vi "Read DAQ Parameters.vi"(8 "error in (no error)":errorcluster, 11 "DAQ Class in":refnum<class "DAQ Class.lvclass">) -> (0 "error out":errorcluster, 2 "DAQ Parameters":T1, 3 "DAQ Class out":refnum<class "DAQ Class.lvclass">)   [LabVIEW 2014, in "DAQ Class.lvclass"]
uses:
  DAQ Class.lvclass
  DAQ Parameters.ctl
  Trigger Source.ctl
  Trigger Slope.ctl
  Type Defs/OCT DAQ Channel Data Type.ctl
  Clock Control.ctl
  DAQ Class.lvclass/DAQ Class.ctl
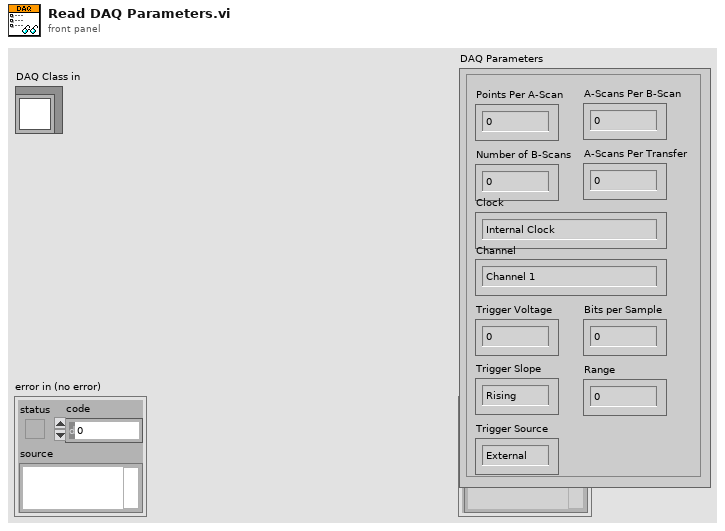
[diagram p1: front panel]
types:
  T1 = typedef "DAQ Class.lvclass/DAQ Parameters.ctl" = cluster{"Points Per A-Scan":u32, "A-Scans Per B-Scan":u32, "Number of B-Scans":u32, "A-Scans Per Transfer":u32, "Trigger Voltage":sgl, "Trigger Source":T2, "Trigger Slope":T3, "Channel":T4, "Clock":T5, "Bits per Sample":dbl, "Range":dbl}
  T2 = typedef "DAQ Class.lvclass/Trigger Source.ctl" = enum16{"External", "Channel A", "Channel B"}
  T3 = typedef "DAQ Class.lvclass/Trigger Slope.ctl" = enum16{"Rising", "Falling"}
  T4 = typedef "OCT DAQ Channel Data Type.ctl" = enum16{"Channel 1", "Channel 2", "Channel 1 and 2"}
  T5 = typedef "DAQ Class.lvclass/Clock Control.ctl" = enum16{"Internal Clock", "External Clock"}
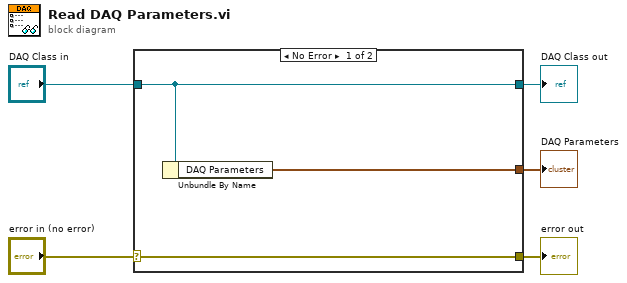
[diagram p0: block diagram]
diagram:
  n1 = case shown="No Error" "error in (no error)" {
    selector: "error in (no error)" -> [w8 w9]
    tunnel: [w8 w9] -> w4
    tunnel: [w7 w10] -> w2
    tunnel: "DAQ Class in" -> [w7 w10]
    tunnel: [w6 _] -> w1
    frame No Error {
      n2 = Unbundle By Name(w7) -> ("DAQ Parameters"=w6:T1)
    }
    frame Error {
    }
  }
  "error out" <- w4
  "DAQ Class out" <- w2
  "DAQ Parameters" <- w1
